vi "Create Builder.vi"(8 "error in (no error)":errorcluster, 10 "File Path Control":path) -> (0 "error out":errorcluster, 3 "CD Build Tools out":refnum<class "Project Build Tools.lvclass">)   [LabVIEW 2019, in "Project Build Tools.lvclass"]
uses:
  Project Build Tools.lvclass
  Project Build Tools.lvclass/Project Build Tools.ctl
panel:
  out "Project Path out":path
  in  "error in (no error) 2":errorcluster
  out "error out 2":errorcluster
  out "Build Specification Names 2":string[](array[string])
  in  "Project Path in":path
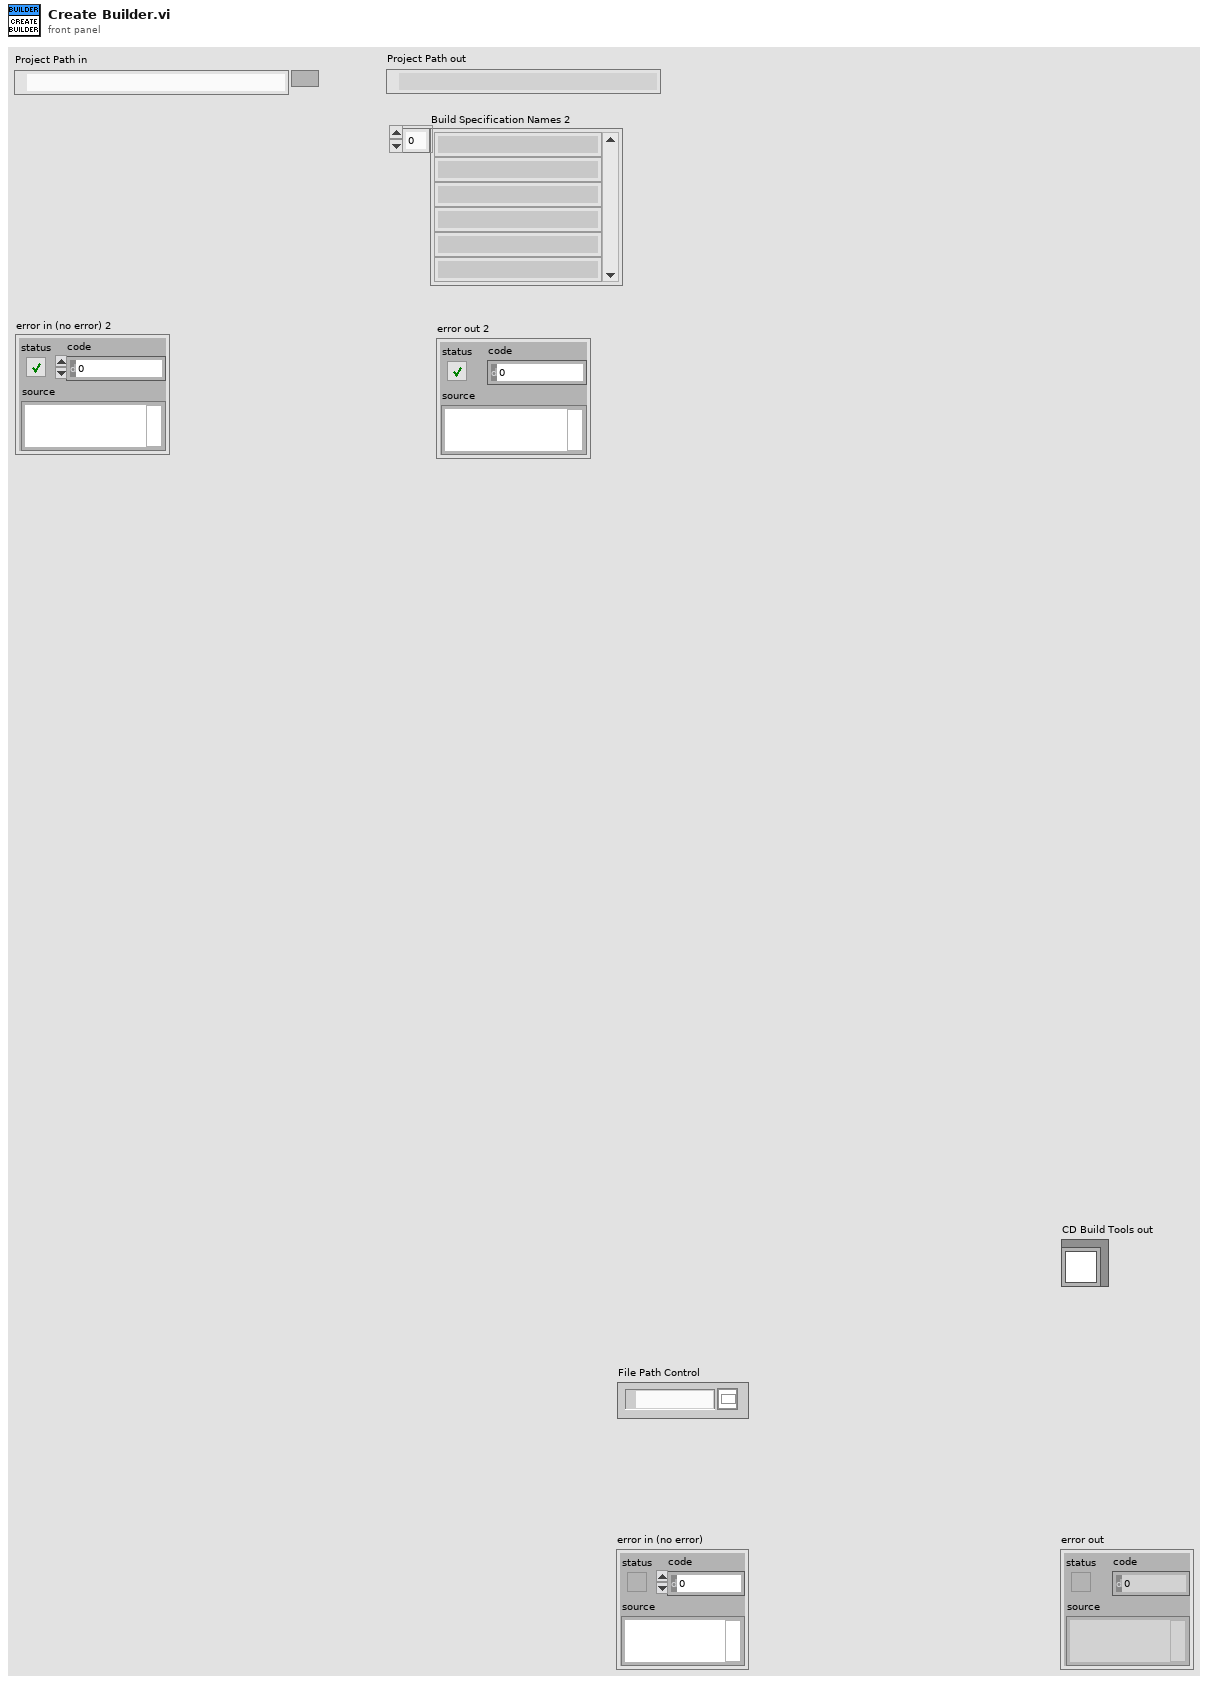
[diagram p1: front panel]
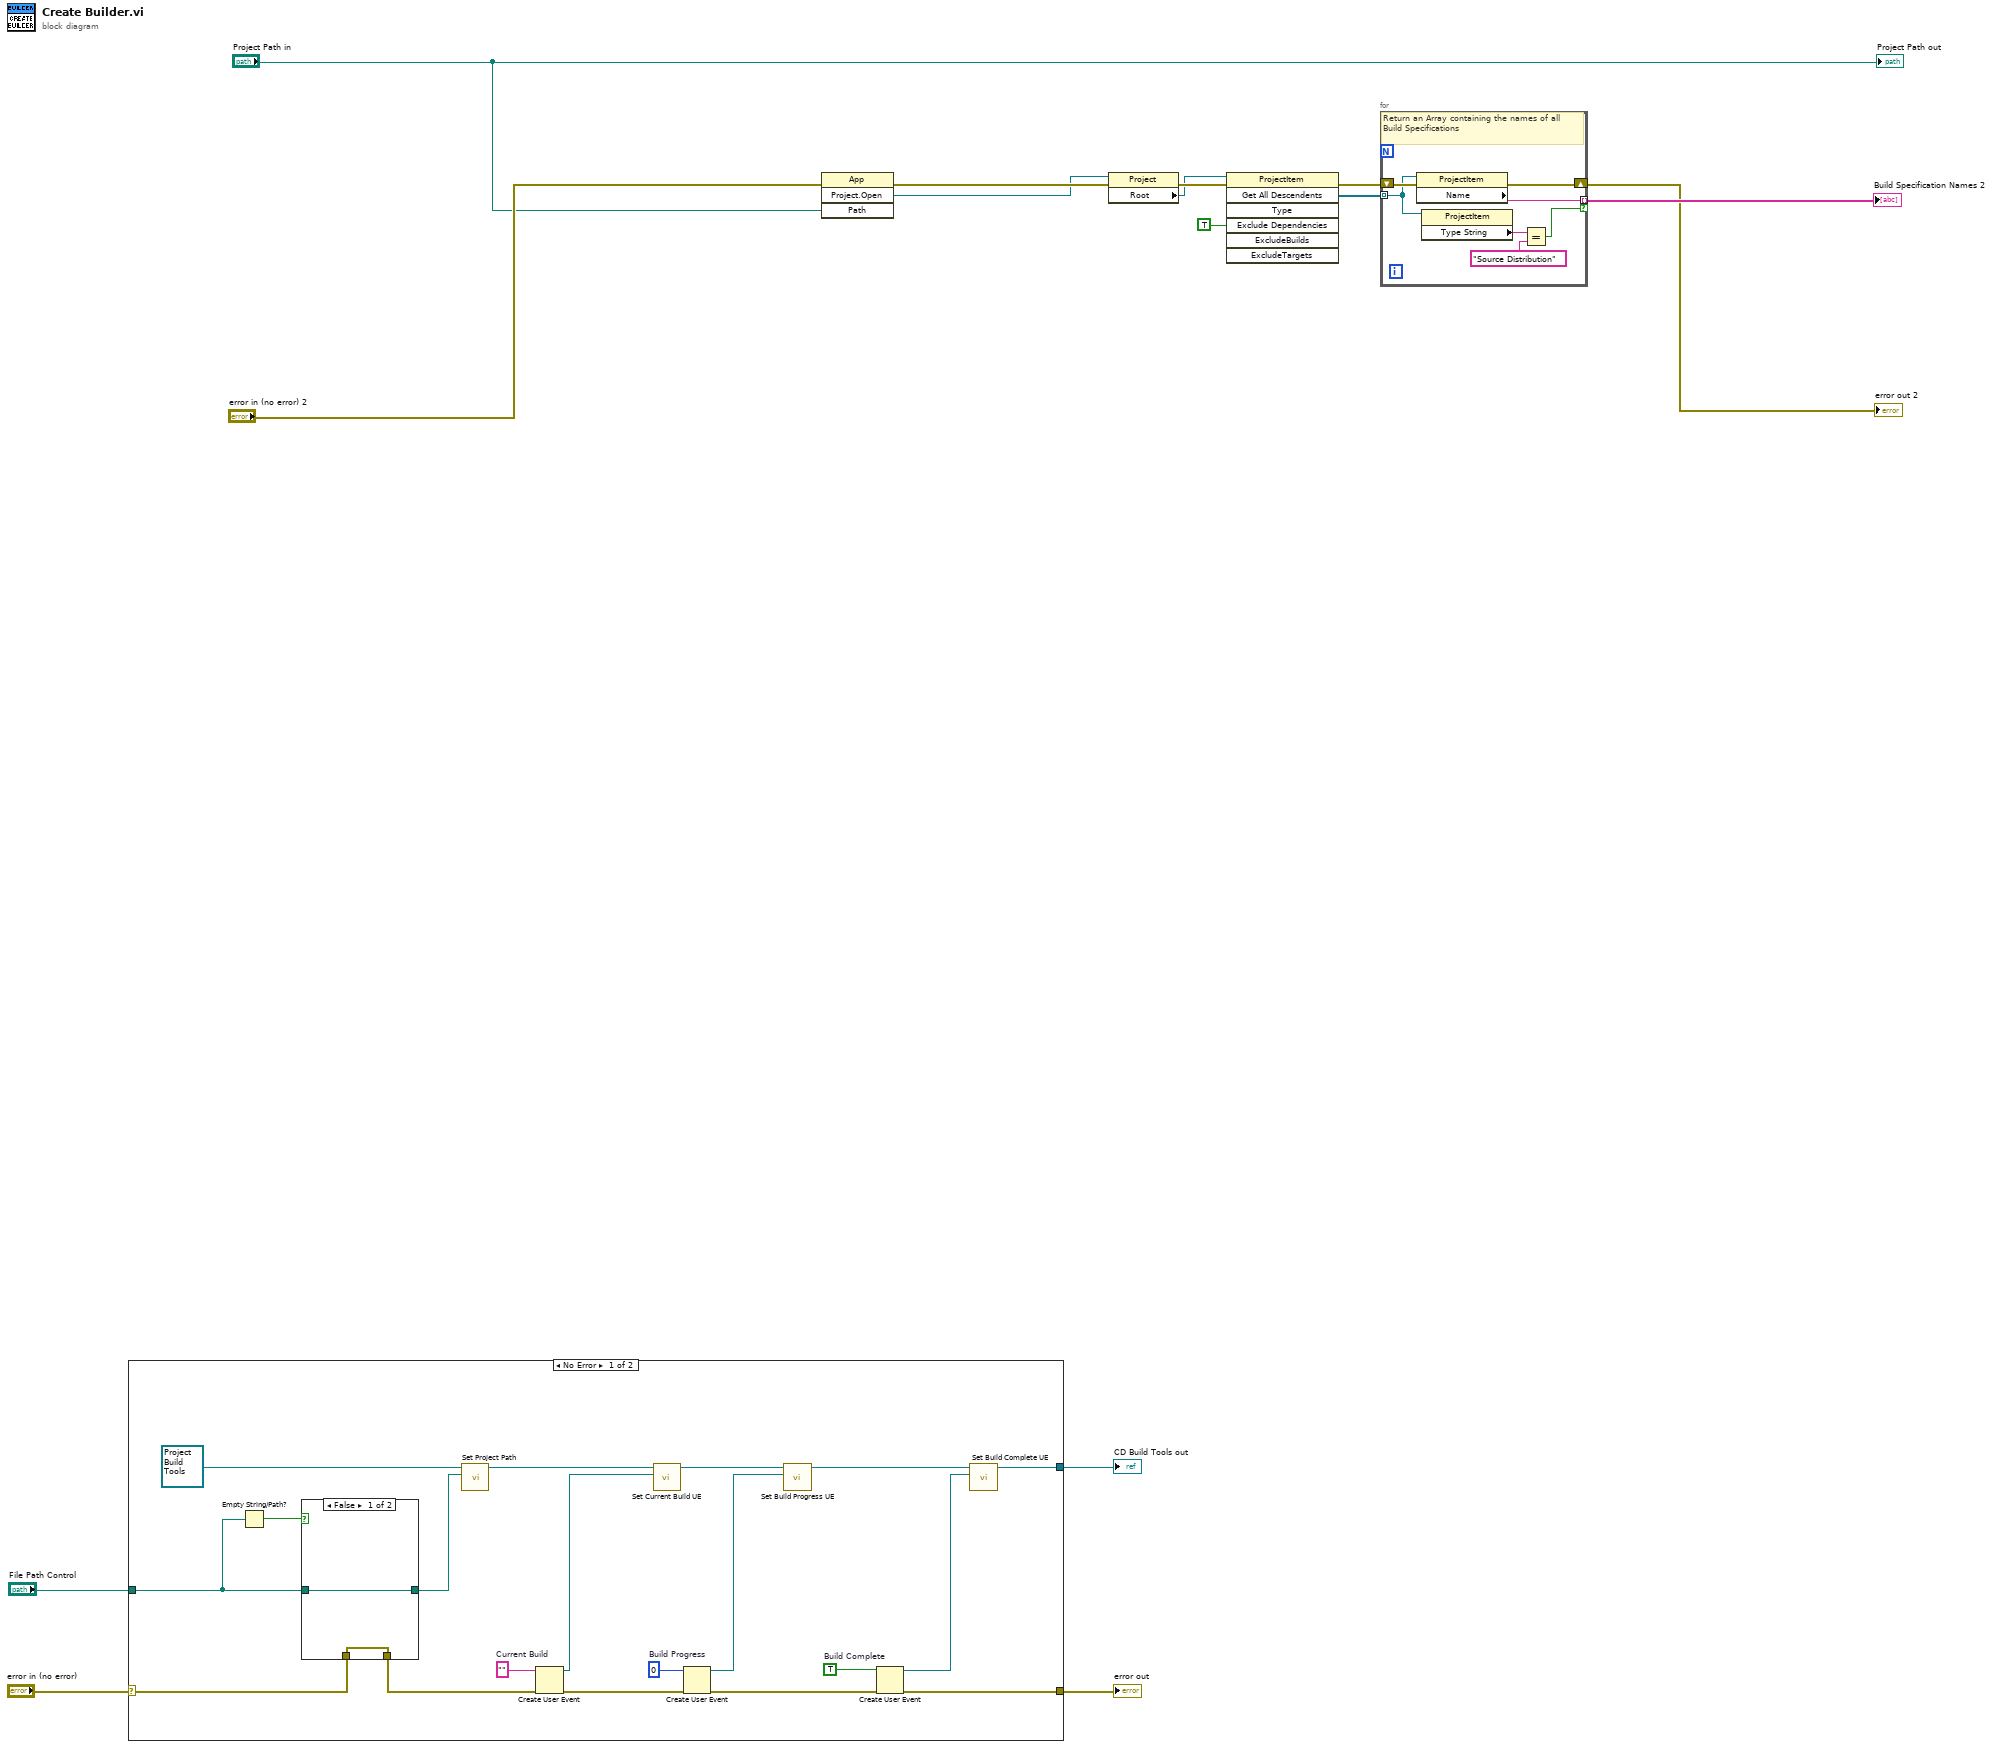
[diagram p0: block diagram]
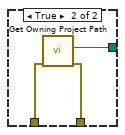
[diagram p2: hidden frame]
diagram:
  n1 = case shown="No Error" "error in (no error)" {
    selector: "error in (no error)" -> [w30 w40]
    tunnel: [w19 w40] -> w14
    tunnel: [w17 _] -> w13
    tunnel: "File Path Control" -> [w32 _]
    frame No Error {
      w21 = TRUE  # Build Complete
      w29 = 0  # Build Progress
      w28 = ""  # Current Build
      n2 = Empty String/Path?(string/path=w32) -> (empty?=w33:bool)
      n3 = case shown="False" w33 {
        tunnel: [w36 w38] -> w31
        tunnel: w32 -> [w36 _]
        tunnel: w30 -> [w35 w39]
        tunnel: [w35 w37] -> w27
        frame False {
        }
        frame True {
          n4 = call "Get Owning Project Path.vi"("error in (no error)"=w39) -> ("error out"=w37:errorcluster, "Path"=w38:path)  [unwired: 9 in]
        }
      }
      n5 = call "Set Project Path.vi"("Project Path"=w31, "CD Build Tools in"=refnum<class "Project Build Tools.lvclass"> refnum ("CD Build Tools out")) -> ("CD Build Tools out"=w24:refnum<class "Project Build Tools.lvclass">)  [unwired: 9 in]
      n6 = Create User Event(user event datatype=w28, error in=w27) -> (user event=w25:refnum<user-event>, error out=w26:errorcluster)
      n7 = call "Set Current Build UE.vi"("Current Build UE"=w25, "CD Build Tools in"=w24) -> ("CD Build Tools out"=w23:refnum<class "Project Build Tools.lvclass">)  [unwired: 9 in]
      n8 = Create User Event(user event datatype=w29, error in=w26) -> (user event=w22:refnum<user-event>, error out=w20:errorcluster)
      n9 = call "Set Build Progress UE.vi"("Build Progress UE"=w22, "CD Build Tools in"=w23) -> ("CD Build Tools out"=w18:refnum<class "Project Build Tools.lvclass">)  [unwired: 9 in]
      n10 = Create User Event(user event datatype=w21, error in=w20) -> (user event=w16:refnum<user-event>, error out=w19:errorcluster)
      n11 = call "Set Build Complete UE.vi"("Build Complete UE"=w16, "CD Build Tools in"=w18) -> ("CD Build Tools out"=w17:refnum<class "Project Build Tools.lvclass">)  [unwired: 9 in]
    }
    frame Error {
    }
  }
  "error out" <- w14
  "CD Build Tools out" <- w13
  n12 = invoke class="App" method="Project.Open"(error in="error in (no error) 2", "Path"="Project Path in") -> (error out=w9:errorcluster, "Project:Open"=w8:refnum<vi>)  [unwired: 2 in, 2 out]
  n13 = property class="Project"(reference=w8, error in=w9) -> (error out=w11:errorcluster, "Root"=w10:refnum<vi>)  [unwired: 1 out]
  n14 = invoke class="ProjectItem" method="Get All Descendents"(reference=w10, error in=w11, "Exclude Dependencies"=TRUE ("ExcludeDependencies")) -> (error out=w6:errorcluster, "All Descendents"=w7:refnum<vi>[])  [unwired: 4 in, 5 out]
  n15 = for {
    tunnel: w7 -> [w44] mode=indexing
    tunnel: [w47] -> w5 mode=indexing if=w41
    shift-right: [w45] -> w3
    shift-left: w6 -> [w46]
    # "Return an Array containing the names of all Build Specifications"
    n16 = property class="ProjectItem"(reference=w44, error in=w46) -> (error out=w45:errorcluster, "Name"=w47:string)  [unwired: 1 out]
    n17 = property class="ProjectItem"(reference=w44) -> ("Type String"=w43:string)  [unwired: 1 in, 2 out]
    n18 = Equal?(x=w43, y="Source Distribution") -> (x = y?=w41:bool)
  }
  "Build Specification Names 2" <- w5
  "error out 2" <- w3
  "Project Path out" <- "Project Path in"
